vi "VNA.Write Configuration File.vi"(8 "error in (no error)":errorcluster, 11 "VNA":refnum<class "VNA.lvclass">) -> (0 "error out":errorcluster, 3 "VNA out":refnum<class "VNA.lvclass">)   [LabVIEW 2016, in "VNA.lvclass"]
uses:
  VNA.lvclass
  C:/Program Files (x86)/National Instruments/LabVIEW 2016/user.lib/LevyLab/Levylab Instruments/SMOs/Instrument/Instrument.lvclass
  <userlib>/LevyLab/Levylab Instruments/SMOs/Instrument/Instrument.lvclass/Instrument.ctl
  VNA.lvclass/VNA.ctl
  <userlib>/LevyLab/Levylab Instruments/SMOs/Configuration/Configuration.lvclass
  <userlib>/LevyLab/Levylab Instruments/SMOs/Instrument/Instrument.lvclass
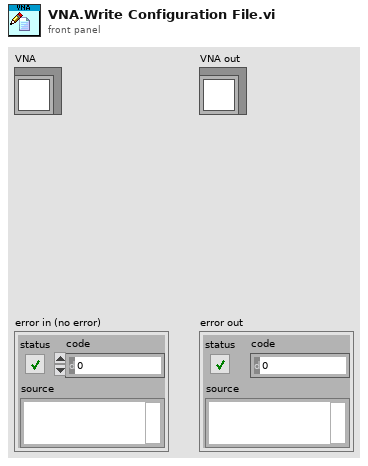
[diagram p1: front panel]
types:
  T1 = typedef "VNA.lvclass/VNA.Configuration--Cluster.ctl" = cluster{"Power":dbl, "Measurement":dbl, "Format":dbl, "Start Freq":dbl, "Stop Freq":dbl, "Num Points":dbl, "Avg Factor":dbl, "Avg?":bool, "Path":path}
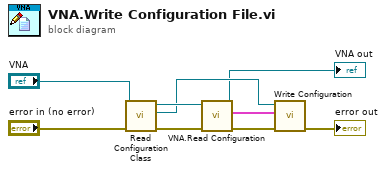
[diagram p0: block diagram]
diagram:
  n1 = call <userlib>:"Read Configuration Class.vi"("error in (no error)"="error in (no error)", "Instrument in"="VNA") -> ("error out"=w5:errorcluster, "Configuration.lvclass"=w8:refnum<class "Configuration.lvclass">, "Instrument out"=w9:refnum<class "VNA.lvclass">)  [unwired: 7 in]
  n2 = call "VNA.Read Configuration.vi"("error in (no error)"=w5, "VNA"=w9) -> ("error out"=w4:errorcluster, "Configuration"=w1:T1, "VNA out"=→"VNA out":refnum<class "VNA.lvclass">)  [unwired: 7 in]
  n3 = call <userlib>:"Write Configuration.vi"("error in (no error)"=w4, "Variant"=w1, "Configuration in"=w8) -> ("error out"=→"error out":errorcluster)  [unwired: 7 in, 1 out]
